vi "ReadMNValuesJSON_EditTolerance_SingleRack.vi"(8 "error in":errorcluster, 11 "JSON file path":path=path "C:/Users/raakeshs/Desktop/ppts/JSON/Write to JSON String/data/Files/test4.json") -> (0 "error out":errorcluster)   [LabVIEW 2015, in "ZenGage v3.0 UI.lvclass"]
uses:
  ZenGage v3.0 UI.lvclass
  Type Definitions/Edit tolerance settings/InputRackController(2Rack).ctl
panel:
  out "InputRackController(2Racks)":T1
  out "Error Message":string
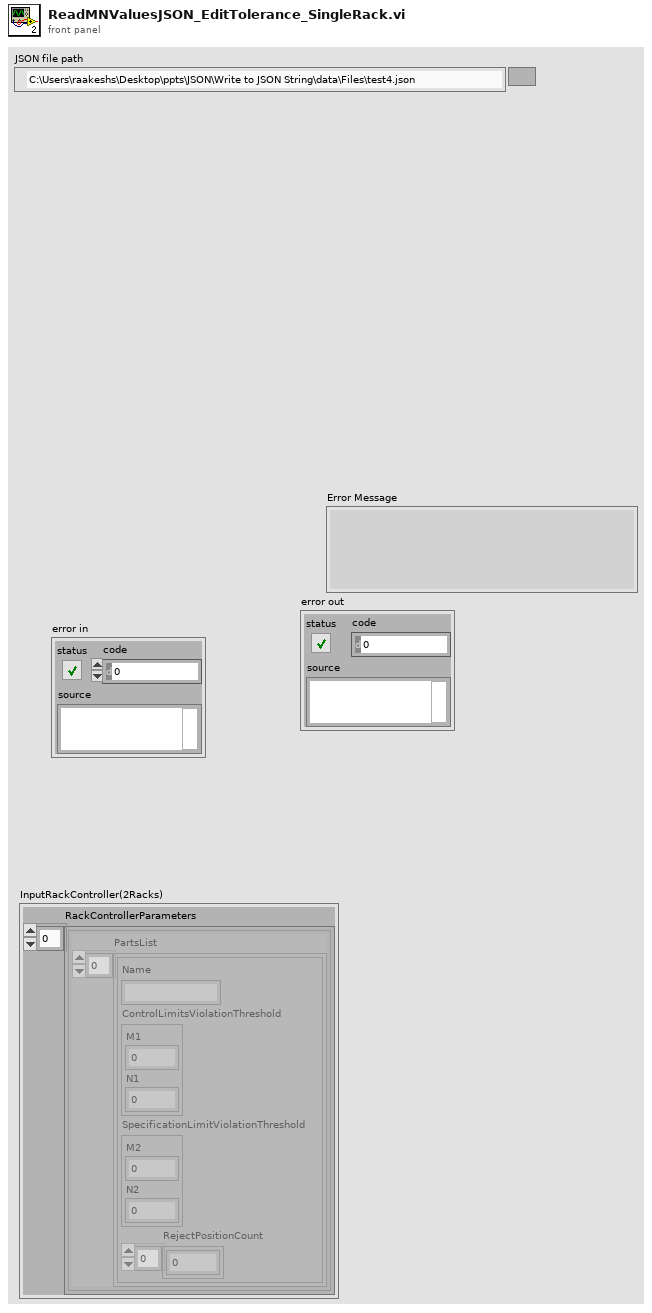
[diagram p1: front panel]
types:
  T1 = typedef "ZenGage v3.0 UI.lvclass/InputRackController(2Rack).ctl" = cluster{"RackControllerParameters":cluster{"PartsList":cluster{"Name":string, "ControlLimitsViolationThreshold":cluster{"M1":i32, "N1":i32}, "SpecificationLimitViolationThreshold":cluster{"M2":i32, "N2":i32}, "RejectPositionCount":i32[]}[]}[]}
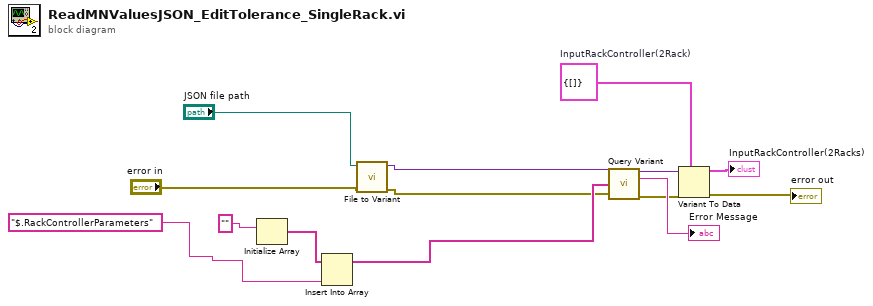
[diagram p0: block diagram]
diagram:
  w6 = T1 {"RackControllerParameters"=[]}  # InputRackController(2Rack)
  n1 = Initialize Array("") -> (w9:string[])  [unwired: 1 in]
  n2 = Insert Into Array(array=w9, new element="$.RackControllerParameters" ("string")) -> (w8:string[])  [unwired: 1 in]
  n3 = call <vilib>:"File to Variant.vi"("JSON FilePath"="JSON file path", "error in (no error)"="error in") -> ("JSON Variant"=w1:variant, "error out"=w3:errorcluster)  [unwired: 6 in, 1 out]
  n4 = call <vilib>:"Query Variant.vi"("VCluster in"=w1, "pathList"=w8, "error IO"=w3) -> ("VCluster\n out"=w13:variant, "Error Message"=→"Error Message":string, "error out"=w12:errorcluster)  [unwired: 9 in, 1 out]
  n5 = Variant To Data(error in=w12, type=w6, Variant=w13) -> (data=→"InputRackController(2Racks)":T1, error out=→"error out":errorcluster)
